vi "ProductDataReadingStringToClusterFormar.vi"(11 "StringFormat":string[](array[string])) -> (3 "ClusterFormat":T1)   [LabVIEW 2014]
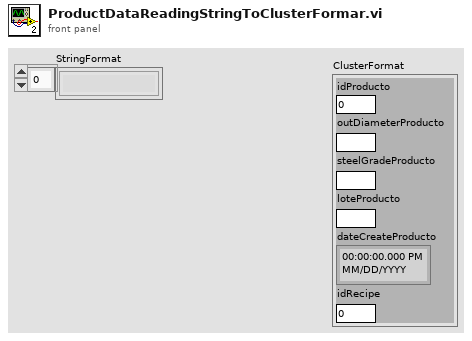
[diagram p1: front panel]
types:
  T1 = cluster{"idProducto":dbl, "outDiameterProducto":string, "steelGradeProducto":string, "loteProducto":string, "dateCreateProducto":timestamp, "idRecipe":dbl}
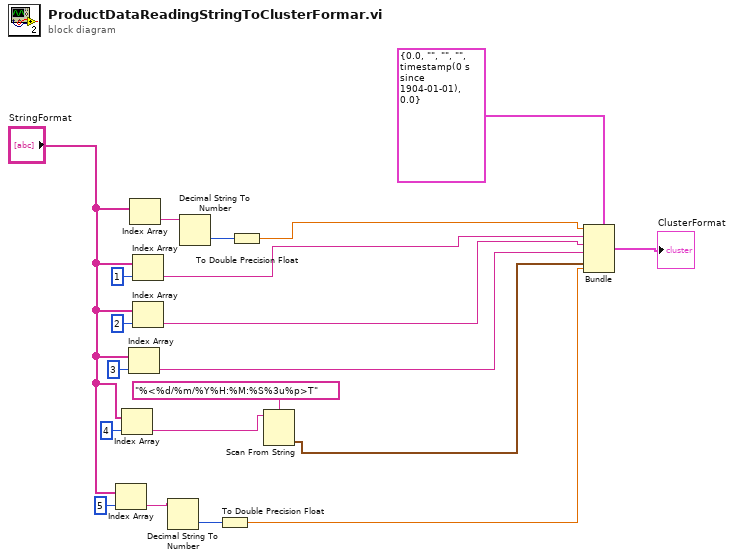
[diagram p0: block diagram]
diagram:
  n1 = Index Array(array="StringFormat", index=5) -> (element=w5:string)
  n2 = Index Array(array="StringFormat", index=4) -> (element=w3:string)
  n3 = Index Array(array="StringFormat", index=3) -> (element=w10:string)
  n4 = Index Array(array="StringFormat") -> (element=w20:string)  [unwired: 1 in]
  n5 = Index Array(array="StringFormat", index=1) -> (element=w13:string)
  n6 = Index Array(array="StringFormat", index=2) -> (element=w12:string)
  n7 = Decimal String To Number(string=w5) -> (number=w6:i32)  [unwired: 2 in, 1 out]
  n8 = Decimal String To Number(string=w20) -> (number=w17:i32)  [unwired: 2 in, 1 out]
  n9 = To Double Precision Float(number=w6) -> (double precision float=w4:dbl)
  n10 = To Double Precision Float(number=w17) -> (double precision float=w14:dbl)
  n11 = Scan From String(format string="%<%d/%m/%Y%H:%M:%S%3u%p>T", input string=w3) -> (output 1=w2:timestamp)  [unwired: 3 in, 3 out]
  n12 = Bundle(cluster=T1 {"idProducto"=0.0, "outDiameterProducto"="", "steelGradeProducto"="", "loteProducto"="", "dateCreateProducto"=timestamp(0 s since 1904-01-01), "idRecipe"=0.0} ("dataToQueryOfRead 2"), "idProducto"=w14, "outDiameterProducto"=w13, "steelGradeProducto"=w12, "loteProducto"=w10, "dateCreateProducto"=w2, "idRecipe"=w4) -> (→"ClusterFormat":T1)
